vi "Verificacion_calibracion.vi"() -> ()   [LabVIEW 2015]
uses:
  <vilib>/LabVIEW Targets/FPGA/cRIO/shared/nicrio_ModuleControls/nicrio_cRIO-9234_DataRatesRing2.ctl
  <vilib>/userDefined/High Color/nirio_resource_hc.ctl
  <vilib>/Analysis/5stat.llb/RMS (DBL).vi
  <vilib>/Analysis/baseanly.llb/Mean (DBL).vi
  <vilib>/FPGAPlugInAG/cRIO-9031/niLvFpga_Open_cRIO-9031.vi
  <vilib>/FPGAPlugInAG/cRIO-9031/niLvFpga_Run_cRIO-9031.vi
  <vilib>/Utility/error.llb/Error Cluster From Error Code.vi
  <vilib>/rvi/errors/niLvFpgaAdjustHostInterfaceError.vi
  <vilib>/rvi/interface/common/niFpgaWaitOnOcc.vi
  <vilib>/FPGAPlugInAG/cRIO-9031/niLvFpga_Reset_cRIO-9031.vi
  <vilib>/measure/madcrms.llb/Basic Averaged DC-RMS for 1 Chan.vi
  <vilib>/measure/maspectr.llb/FFT Spectrum (Mag-Phase) for 1 Chan.vi
  <vilib>/FPGAPlugInAG/cRIO-9031/niLvFpga_Close_cRIO-9031.vi
  <vilib>/rvi/interface/nirviOpenFPGA/nirviOpenFPGA.xnode
  FPGA Bitfiles/W&RDEuskotrenIBA_FPGATarget2_FPGA8a2wsBIdirec_MwruJOs6jio.lvbitx
  <vilib>/rvi/interface/nirviMethod/nirviMethod.xnode
  <vilib>/rvi/interface/nirviReadWriteControl/nirviReadWriteControl.xnode
  <vilib>/rvi/interface/nirviCloseFPGA/nirviCloseFPGA.xnode
  <vilib>/measure/NI_MAPro.lvlib
  <vilib>/Analysis/NI_AALPro.lvlib
  <vilib>/Analysis/NI_AALBase.lvlib
  NiFpgaLv.dll
  <vilib>/rvi/errors/niLvFpgaMergeErrorWithErrorCode.vi
  <vilib>/FPGAPlugInAG/cRIO-9031/niLvFpga_ConfigureFifo_cRIO-9031.vi
  <vilib>/FPGAPlugInAG/cRIO-9031/niLvFpga_StartFifo_cRIO-9031.vi
  <vilib>/FPGAPlugInAG/cRIO-9031/niLvFpga_ReadFifo_cRIO-9031.vi
  <vilib>/FPGAPlugInAG/cRIO-9031/niLvFpga_StopFifo_cRIO-9031.vi
panel:
  in  "Aceleración del patrón (g RMS)":dbl=1.0
  in  "Frecuencia del patrón (Hz)":dbl=159.2
  out "RMS conseguido":dbl format="%0.2f"
  in  "Data Rate":T1=2 items=["51.200 kS/s (NI 9234)"=1, "25.600 kS/s (NI 9234)"=2, "17.067 kS/s (NI 9234)"=3, "12.800 kS/s (NI 9234)"=4, "10.240 kS/s (NI 9234)"=5, "8.533 kS/s (NI 9234)"=6, "7.314 kS/s (NI 9234)"=7, "6.400 kS/s (NI 9234)"=8, "5.689 kS/s (NI 9234)"=9, "5.120 kS/s (NI 9234)"=10, "4.654 kS/s (NI 9234)"=11, "4.267 kS/s (NI 9234)"=12, "3.938 kS/s (NI 9234)"=13, "3.657 kS/s (NI 9234)"=14, "3.413 kS/s (NI 9234)"=15, "3.200 kS/s (NI 9234)"=16, "3.012 kS/s (NI 9234)"=17, "2.845 kS/s (NI 9234)"=18, "2.695 kS/s (NI 9234)"=19, "2.560 kS/s (NI 9234)"=20, "2.438 kS/s (NI 9234)"=21, "2.328 kS/s (NI 9234)"=22, "2.226 kS/s (NI 9234)"=23, "2.133 kS/s (NI 9234)"=24, "2.048 kS/s (NI 9234)"=25, "1.969 kS/s (NI 9234)"=26, "1.896 kS/s (NI 9234)"=27, "1.829 kS/s (NI 9234)"=28, "1.765 kS/s (NI 9234)"=29, "1.707 kS/s (NI 9234)"=30, "1.652 kS/s (NI 9234)"=31]
  in  "Nº del canal":i32
  out "Waveform Graph 2":cluster{"f0":dbl, "df":dbl, "magnitude":dbl[]}(graph)
  out "error out":errorcluster
  out "Chassis \nTemperature":i16
  in  "Adquirir":bool
  out "Waveform Graph":waveform(dbl)[](graph)
  out "Frecuencia de excitación\nVibrómetro  (Hz)":dbl
  in  "Parámetro de sensibilidad\n           (mV/g)":sgl=10.0
  in  "Frecuencia de muestreo (Hz)":dbl=25600.0
  in  "Canales a calibrar (4 o 8)":u32=8
  out "Nombre de archivo":path
  out "Tiempo de paso (s)":dbl
  in  "Tiempo de adquisición":dbl=1.0
  out "Buffer Overflow":bool
  out "Buffer Underflow":bool
  in  "stop":bool
  out "Inicio pasada":timestamp
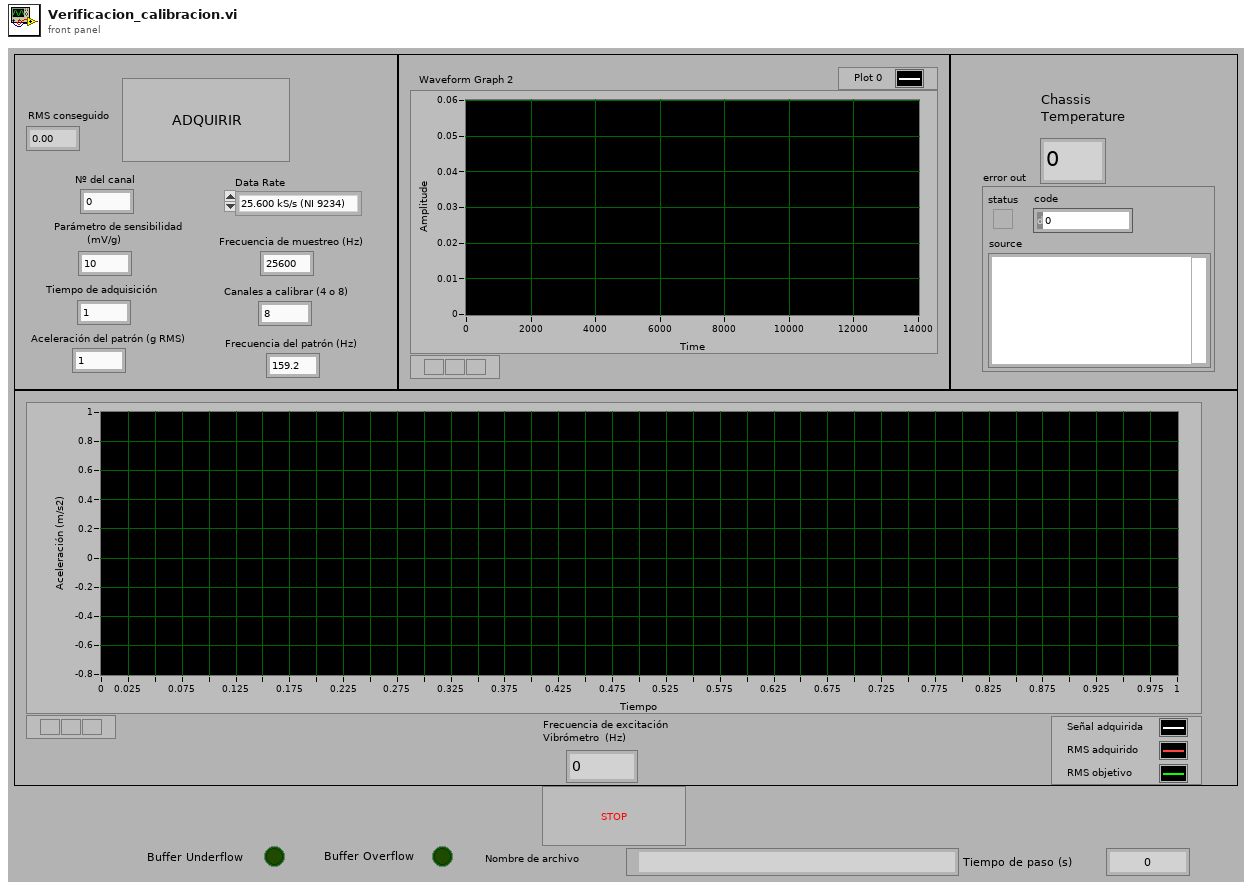
[diagram p1: front panel]
types:
  T1 = typedef "nicrio_cRIO-9234_DataRatesRing2.ctl" = u8
  T2 = typedef "nirio_resource_hc.ctl" = tag
  T3 = enum16{"open", "replace", "create", "open or create", "replace or create", "replace or create with confirmation"}
  T4 = enum16{"big-endian, network order", "native, host order", "little-endian"}
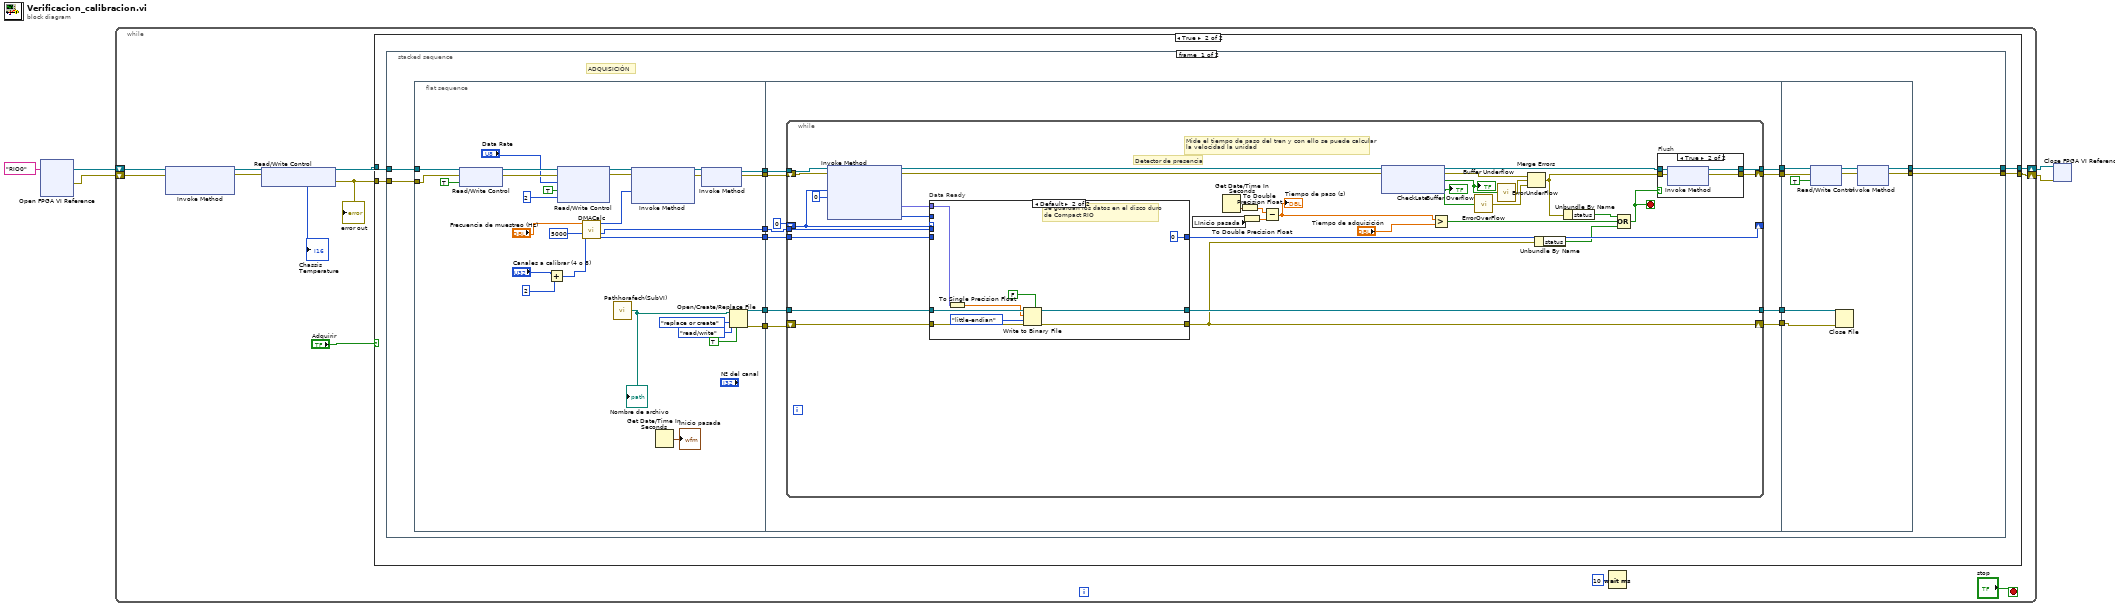
[diagram p0: block diagram]
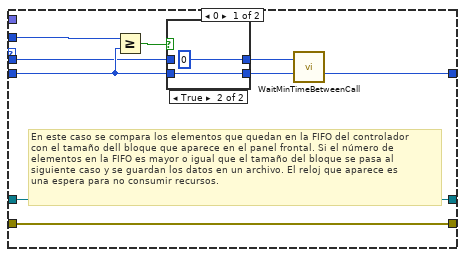
[diagram p3: hidden frame]
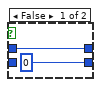
[diagram p4: hidden frame]
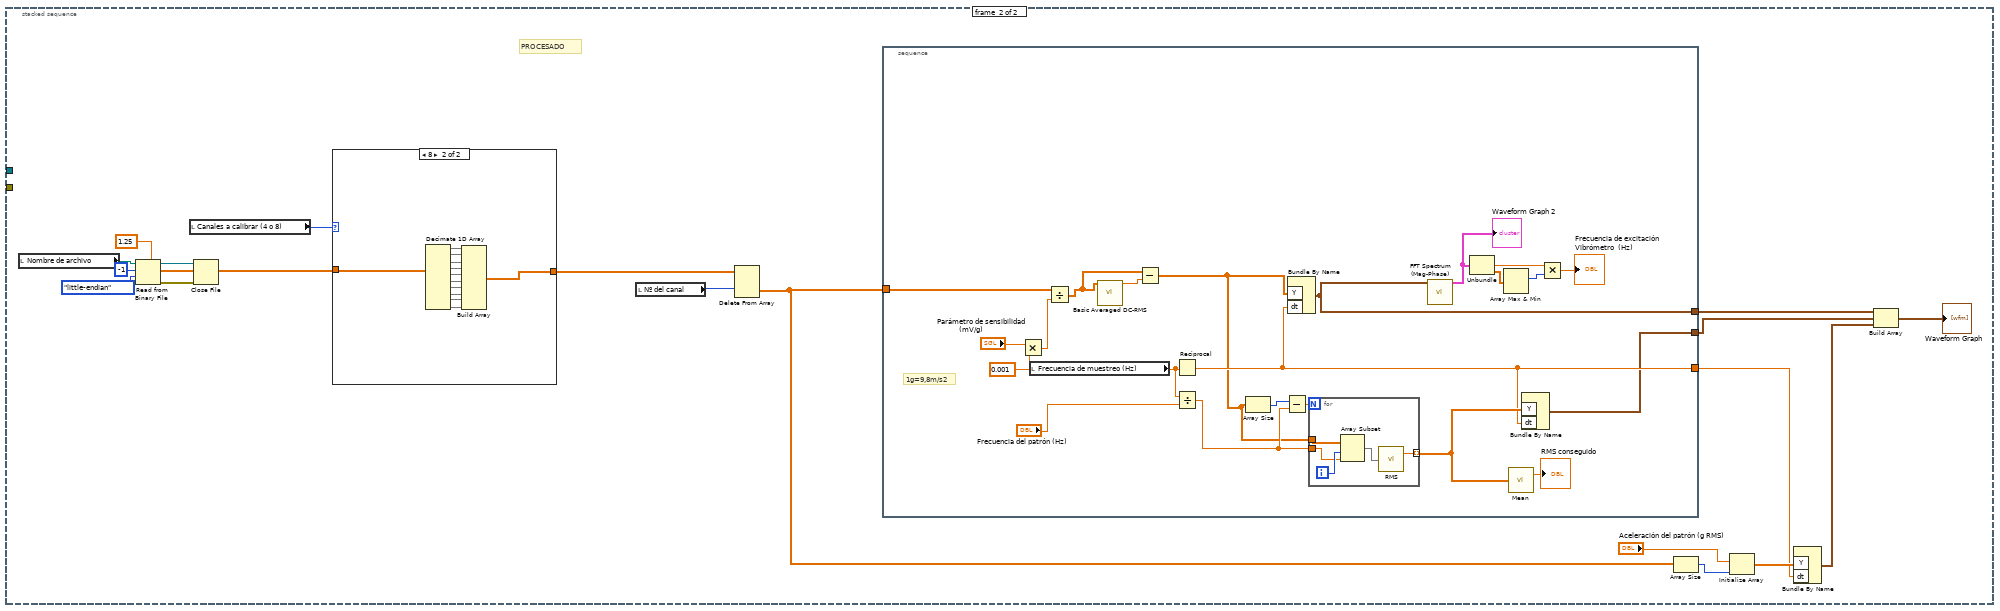
[diagram p6: hidden frame]
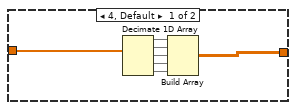
[diagram p7: hidden frame]
diagram:
  n1 = xnode "Open FPGA VI Reference"("resource name"=T2 "RIO0") -> ("FPGA VI Reference Out"=w5:refnum<k20>, "error out"=w2:errorcluster)  [unwired: 1 in]
  n2 = while {
    shift-right: [w10] -> w3
    shift-left: w5 -> [w8]
    shift-right: [w15] -> w4
    shift-left: w2 -> [w7]
    stop <- "stop" stop-if-true
    n3 = xnode "Invoke Method"("FPGA VI Reference In"=w8, "error in"=w7) -> ("FPGA VI Reference Out"=w9:refnum<k20>, "error out"=w6:errorcluster)  [unwired: 1 in]
    n4 = xnode "Read/Write Control"("FPGA VI Reference In"=w9, "error in"=w6) -> ("FPGA VI Reference Out"=w13:refnum<k20>, "error out"=w12:errorcluster, "Chassis Temperature"=→"Chassis \nTemperature":i16)
    "error out" <- w12
    n5 = case shown="True" "Adquirir" {
      tunnel: w13 -> [w19 w23]
      tunnel: w12 -> [w18 w22]
      tunnel: [w19 w21] -> w10
      tunnel: [w18 w20] -> w15
      frame False {
      }
      frame True {
        n6 = stacked-sequence {
          tunnel: w23 -> [w27 _]
          tunnel: w22 -> [w26 _]
          tunnel: [w25 _] -> w21
          tunnel: [w24 _] -> w20
          frame #0 {
            # "ADQUISICIÓN"
            n7 = flat-sequence {
              tunnel: w26 -> [w47]
              tunnel: w27 -> [w48]
              tunnel: [w59] -> w37
              tunnel: [w58] -> w36
              tunnel: [w57] -> w35
              tunnel: [w56] -> w34
              tunnel: [w55] -> w33
              tunnel: [w54] -> w32
              tunnel: [w76] -> w31
              tunnel: [w75] -> w30
              tunnel: [w74] -> w29
              tunnel: [w67] -> w28
              tunnel: w37 -> [w73]
              tunnel: w36 -> [w72]
              tunnel: w35 -> [w71]
              tunnel: w34 -> [w70]
              tunnel: w33 -> [w69]
              tunnel: w32 -> [w68]
              tunnel: w31 -> [w143]
              tunnel: w30 -> [w142]
              tunnel: w29 -> [w145]
              tunnel: w28 -> [w144]
              tunnel: [w146] -> w24
              tunnel: [w147] -> w25
              frame #0 {
                n8 = xnode "Read/Write Control"("FPGA VI Reference In"=w48, "error in"=w47, "Fotocélula"=TRUE ("Adquirir")) -> ("FPGA VI Reference Out"=w46:refnum<k20>, "error out"=w45:errorcluster)
                n9 = Add(x="Canales a calibrar (4 o 8)", y=u32 2) -> (x+y=w39:u32)
                n10 = xnode "Read/Write Control"("FPGA VI Reference In"=w46, "error in"=w45, "Data Rate"="Data Rate", "Digital?"=TRUE, "Count(mSec)"=u32 2) -> ("FPGA VI Reference Out"=w52:refnum<k20>, "error out"=w51:errorcluster)
                n11 = call "DMACalc.vi"("Number of Channels"=w39, "Number of Samples"=u32 5000, "Rate (Hz)"="Frecuencia de muestreo (Hz)") -> ("Block Size"=w56:u32, "Time to Acquire Block (ms)"=w57:i32, "Host Buffer Size"=w61:u32)  [unwired: 6 in]
                n12 = call "Pathhorafech(SubVI).vi"() -> ("path"=w60:path)
                "Nombre de archivo" <- w60
                n13 = xnode "Invoke Method"("FPGA VI Reference In"=w52, "error in"=w51, "Requested Depth"=w61) -> ("FPGA VI Reference Out"=w63:refnum<k20>, "error out"=w62:errorcluster)  [unwired: 1 out]
                n14 = Get Date/Time In Seconds() -> (seconds since 1Jan1904=→"Inicio pasada":timestamp)
                n15 = xnode "Invoke Method"("FPGA VI Reference In"=w63, "error in"=w62) -> ("FPGA VI Reference Out"=w59:refnum<k20>, "error out"=w58:errorcluster)
                n16 = Open/Create/Replace File(file path (use dialog)=w60, operation (0:open)=T3."replace or create", access (0:read/write)=enum16{"read/write", "read-only", "write-only"}."read/write", disable buffering (F)=TRUE) -> (refnum out=w55:refnum<file>, error out=w54:errorcluster)  [unwired: 1 in, 2 out]
              }
              frame #1 {
                n17 = while "Data Acquisition" {
                  tunnel: w73 -> [w102]
                  shift-right: [w109] -> _
                  shift-left: u32 0 ("t") -> [w105]
                  tunnel: w71 -> [w110]
                  tunnel: w70 -> [w108]
                  shift-right: [w111] -> w75
                  shift-left: w72 -> [w101]
                  tunnel: [w106] -> w76
                  tunnel: w69 -> [w89]
                  tunnel: [w90] -> w74
                  shift-right: [w88] -> w67
                  shift-left: w68 -> [w99]
                  stop <- w107 stop-if-true
                  # "Detector de presencia"
                  # "Mide el tiempo de paso del tren y con ello se puede calcular\nla velocidad la unidad"
                  n18 = xnode "Invoke Method"("FPGA VI Reference In"=w102, "error in"=w101, "Number of Elements"=w105, "Timeout (ms)"=0) -> ("FPGA VI Reference Out"=w87:refnum<k20>, "error out"=w86:errorcluster, "Data"=w100:fxp<+/-,24,4>[], "Elements Remaining"=w103:u32)
                  n19 = case "Data Ready" shown="Default" w105 {
                    tunnel: w110 -> [w116 _]
                    tunnel: [w115 u32 0 ("t")] -> w109
                    tunnel: w108 -> [w117 _]
                    tunnel: w103 -> [w114 _]
                    tunnel: w100 -> [_ w127]
                    tunnel: w99 -> [w113 w129]
                    tunnel: [w113 w128] -> w88
                    tunnel: w89 -> [w112 w126]
                    tunnel: [w112 w125] -> w90
                    frame 0 {
                      # "En este caso se compara los elementos que quedan en la FIFO del controlador\ncon el tamaño dell bloque que aparece en el panel frontal. Si el número de\nelementos en la FIFO es mayor o igual que el tamaño del bloque se pasa al\nsiguiente caso y se guardan los datos en un archivo. El reloj que aparece es\nuna espera para no consumir recursos."
                      n20 = Greater Or Equal?(x=w114, y=w117) -> (x >= y?=w118:bool)
                      n21 = case shown="True" w118 {
                        tunnel: [u32 0 ("Block Size") w122] -> w115
                        tunnel: [w121 0 ("t")] -> w119
                        tunnel: w116 -> [w121 _]
                        tunnel: w117 -> [_ w122]
                        frame False {
                        }
                        frame True {
                        }
                      }
                      n22 = call "WaitMinTimeBetweenCall.vi"("Minimum ms between calls"=w119) -> ()  [unwired: 2 in]
                    }
                    frame Default {
                      # "Se guardan los datos en el disco duro\nde Compact RIO"
                      n23 = To Single Precision Float(number=w127) -> (single precision float=w124:sgl[])
                      n24 = Write to Binary File(file (use dialog)=w126, data=w124, error in=w129, 5:FALSE ("prepend array or string size? (T)"), 9:T4."little-endian" ("byte order (0:big-endian, network order)")) -> (refnum out=w125:refnum<file>, error out=w128:errorcluster)  [unwired: 2 out]
                    }
                  }
                  n25 = local read "Inicio pasada"() -> (w84:timestamp)
                  n26 = Get Date/Time In Seconds() -> (seconds since 1Jan1904=w83:timestamp)
                  n27 = To Double Precision Float(number=w83) -> (double precision float=w81:dbl)
                  n28 = To Double Precision Float(number=w84) -> (double precision float=w85:dbl)
                  n29 = Subtract(x=w81, y=w85) -> (x-y=w92:dbl)
                  "Tiempo de paso (s)" <- w92
                  n30 = xnode ("CheckLate")("FPGA VI Reference In"=w87, "error in"=w86) -> ("FPGA VI Reference Out"=w78:refnum<k20>, "error out"=w95:errorcluster, "Buffer Underflow"=w96:bool, "Buffer Overflow"=w97:bool)
                  "Buffer Underflow" <- w96
                  "Buffer Overflow" <- w97
                  n31 = Greater?(x=w92, y="Tiempo de adquisición") -> (0:w80:bool)
                  n32 = call "ErrorOverFlow.vi"("Buffer Overflow"=w97) -> ("error out"=w93:errorcluster)
                  n33 = call "ErrorUnderFlow.vi"("Buffer Overflow"=w96) -> ("error out"=w94:errorcluster)
                  n34 = Merge Errors(w95, w94, w93) -> (w79:errorcluster)
                  n35 = Unbundle By Name(w88) -> ("status"=w91:bool)
                  n36 = Unbundle By Name(w79) -> ("status"=w98:bool)
                  n37 = Compound Arithmetic op=OR(w98, w80, w91) -> (w107:bool)
                  n38 = case "Flush" shown="True" w107 {
                    tunnel: w78 -> [w133 w138]
                    tunnel: w79 -> [w134 w137]
                    tunnel: [w134 w136] -> w111
                    tunnel: [w133 w135] -> w106
                    frame False {
                    }
                    frame True {
                      n39 = xnode "Invoke Method"("FPGA VI Reference In"=w138, "error in"=w137) -> ("FPGA VI Reference Out"=w135:refnum<k20>, "error out"=w136:errorcluster)
                    }
                  }
                }
              }
              frame #2 {
                n40 = xnode "Read/Write Control"("FPGA VI Reference In"=w143, "error in"=w142, "Stop"=TRUE ("stop")) -> ("FPGA VI Reference Out"=w141:refnum<k20>, "error out"=w140:errorcluster)
                n41 = Close File(refnum=w145, error in=w144) -> ()  [unwired: 2 out]
                n42 = xnode "Invoke Method"("FPGA VI Reference In"=w141, "error in"=w140) -> ("FPGA VI Reference Out"=w147:refnum<k20>, "error out"=w146:errorcluster)
              }
            }
          }
          frame #1 {
            # "PROCESADO"
            n43 = local read "Nombre de archivo"() -> (w163:path)
            n44 = Read from Binary File(5:sgl 1.25, 9:T4."little-endian" ("byte order (0:big-endian, network order)"), 10:-1 ("count (1)"), 11:w163) -> (0:w166:errorcluster, 2:w159:sgl[], 3:w162:refnum<file>)  [unwired: 1 in, 2 out]
            n45 = local read "Canales a calibrar (4 o 8)"() -> (w160:u32)
            n46 = Close File(refnum=w162, error in=w166) -> ()  [unwired: 2 out]
            n47 = case shown="8" w160 {
              tunnel: w159 -> [w197 w209]
              tunnel: [w196 w208] -> w158
              frame 4, Default {
                n48 = Decimate 1D Array(w197) -> (w199:sgl[], w200:sgl[], w198:sgl[], w195:sgl[], w194:sgl[])
                n49 = Build Array(w199, w200, w198, w195, w194) -> (w196:sgl[][])
              }
              frame 8 {
                n50 = Decimate 1D Array(w209) -> (w211:sgl[], w212:sgl[], w210:sgl[], w204:sgl[], w203:sgl[], w205:sgl[], w206:sgl[], w207:sgl[], w202:sgl[], w201:sgl[])
                n51 = Build Array(w211, w212, w210, w204, w203, w205, w206, w207, w202, w201) -> (w208:sgl[][])
              }
            }
            n52 = local read "Nº del canal"() -> (w157:i32)
            n53 = Delete From Array(array=w158, index (row)=w157) -> (deleted portion=w151:sgl[])  [unwired: 2 in, 1 out]
            n54 = stacked-sequence {
              tunnel: [w181] -> w156
              tunnel: [w169] -> w153
              tunnel: w151 -> [w178]
              tunnel: [w167] -> w148
              frame #0 {
                # "1g=9,8m/s2"
                n55 = Multiply(x="Parámetro de sensibilidad\n           (mV/g)", y=0.001) -> (x*y=w183:dbl)
                n56 = local read "Frecuencia de muestreo (Hz)"() -> (w171:dbl)
                n57 = Divide(x=w178, y=w183) -> (x/y=w177:dbl[])
                n58 = call-poly <vilib>:"Basic Averaged DC-RMS.vi"("signal in"=w177) -> ("DC value"=w180:dbl)  [unwired: 7 in, 3 out]
                n59 = Subtract(x=w177, y=w180) -> (x-y=w168:dbl[])
                n60 = Reciprocal(x=w171) -> (1/x=w169:dbl)
                n61 = Divide(x=w171, y="Frecuencia del patrón (Hz)") -> (x/y=w174:dbl)
                n62 = Array Size(array=w168) -> (size(s)=w175:i32)
                n63 = Subtract(x=w175, y=w174) -> (x-y=w176:dbl)
                n64 = Bundle By Name("Y"=w168, "dt"=w169) -> (w181:waveform(dbl))  [unwired: 1 in]
                n65 = for {
                  N: w176 -> [_]
                  tunnel: w174 -> [w190]
                  tunnel: [w193] -> w173 mode=indexing
                  tunnel: w168 -> [w192]
                  i -> [w191]
                  n66 = Array Subset(array=w192, index=w191, length=w190) -> (w189:dbl[])
                  n67 = call-poly <vilib>:"RMS.vi"("X"=w189) -> ("rms value"=w193:dbl)  [unwired: 1 out]
                }
                n68 = call-poly <vilib>:"FFT Spectrum (Mag-Phase).vi"("time signal"=w181) -> ("magnitude"=w184:cluster{"f0":dbl, "df":dbl, "magnitude":dbl[]})  [unwired: 6 in, 4 out]
                "Waveform Graph 2" <- w184
                n69 = Unbundle(w184) -> ("df"=w186:dbl, "magnitude"=w187:dbl[])  [unwired: 1 out]
                n70 = Array Max & Min(array=w187) -> (max index (indices)=w188:i32)  [unwired: 3 out]
                n71 = call-poly <vilib>:"Mean.vi"("X"=w173) -> ("mean"=→"RMS conseguido":dbl)  [unwired: 1 out]
                n72 = Bundle By Name("Y"=w173, "dt"=w169) -> (w167:waveform(dbl))  [unwired: 1 in]
                n73 = Multiply(x=w186, y=w188) -> (x*y=→"Frecuencia de excitación\nVibrómetro  (Hz)":dbl)
              }
            }
            n74 = Array Size(array=w151) -> (size(s)=w155:i32)
            n75 = Initialize Array("Aceleración del patrón (g RMS)", w155) -> (w154:dbl[])
            n76 = Bundle By Name("Y"=w154, "dt"=w153) -> (w150:waveform(dbl))  [unwired: 1 in]
            n77 = Build Array(w156, w148, w150) -> (→"Waveform Graph":waveform(dbl)[])
          }
        }
      }
    }
    n78 = Wait (ms)(milliseconds to wait=u32 10) -> ()  [unwired: 1 out]
  }
  n79 = xnode "Close FPGA VI Reference"("FPGA VI Reference In"=w3, "error in"=w4) -> ()  [unwired: 1 out]
